vi "ZNA_setMarker.vi"(5 "Step_Freq(GHz)":dbl=0.5 format="%#_13g", 7 "Start_Freq(GHz)":dbl=26.5 format="%#_13g", 8 "error in":errorcluster, 9 "Simulation":bool, 10 "Markers_num":i32=11, 11 "VISA IN":refnum<visa-resource-name>="TCPIP0::192.168.100.12::inst0::INSTR") -> (0 "error out":errorcluster, 3 "Marker_array":dbl[](array[numeric]))   [LabVIEW 2023, in "R_S.lvlib"]
uses:
  R_S.lvlib
  CTL/RS_ZNA.ctl
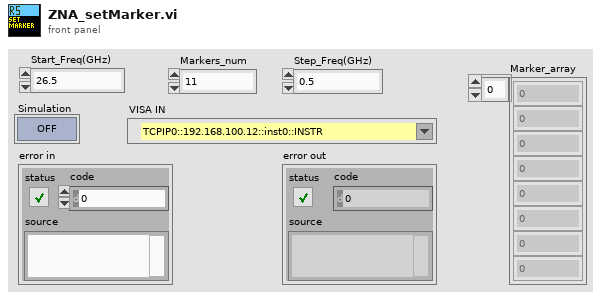
[diagram p1: front panel]
types:
  T1 = typedef "RS_ZNA.ctl" = enum16{"Init", "Close", "set_SweepPoint", "set_MeasFormat", "set_FreqStartStop", "set_MeasPAR_S", "set_MarkerON", "set_MarkerOFF", "set_MarkerFreq", "set_MarkerFormat", "set_TriggerSingle", "query_GainPhase"}
  T2 = cluster{"SweepPoints":i32, "StartFreq_GHz":dbl, "StopFreq_GHz":dbl, "S_Parameter":i32, "Marker_no.":i32, "Marker_Freq(GHz)":dbl}
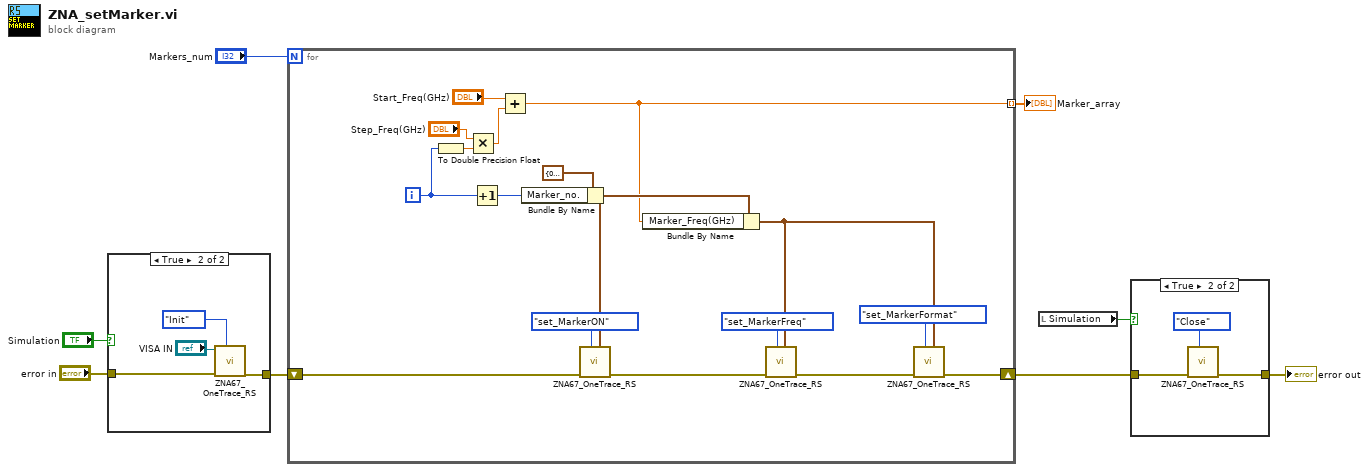
[diagram p0: block diagram]
diagram:
  n1 = case shown="True" "Simulation" {
    tunnel: "error in" -> [w9 w13]
    tunnel: [w9 w11] -> w7
    frame False {
    }
    frame True {
      n2 = call "ZNA67_OneTrace_RS.vi"("ZNA_Func."=RS_ZNA."Init", "error in"=w13, "VISA IN"="VISA IN") -> ("error out"=w11:errorcluster)  [unwired: 5 in, 3 out]
    }
  }
  n3 = for {
    N: "Markers_num" -> [_]
    shift-right: [w20] -> w6
    shift-left: w7 -> [w30]
    tunnel: [w18] -> w1 mode=indexing
    i -> [w28]
    n4 = To Double Precision Float(number=w28) -> (double precision float=w26:dbl)
    n5 = Multiply(x="Step_Freq(GHz)", y=w26) -> (x*y=w24:dbl)
    n6 = Increment(x=w28) -> (x+1=w22:i32)
    n7 = Add(x="Start_Freq(GHz)", y=w24) -> (x+y=w18:dbl)
    n8 = Bundle By Name(cluster=T2 {"SweepPoints"=0, "StartFreq_GHz"=0.0, "StopFreq_GHz"=0.0, "S_Parameter"=0, "Marker_no."=0, "Marker_Freq(GHz)"=0.0} ("ZNA_Parameters"), "Marker_no."=w22) -> (w23:T2)
    n9 = call "ZNA67_OneTrace_RS.vi"("ZNA_Parameters"=w23, "ZNA_Func."=RS_ZNA."set_MarkerON", "error in"=w30) -> ("error out"=w29:errorcluster)  [unwired: 5 in, 3 out]
    n10 = Bundle By Name(cluster=w23, "Marker_Freq(GHz)"=w18) -> (w19:T2)
    n11 = call "ZNA67_OneTrace_RS.vi"("ZNA_Parameters"=w19, "ZNA_Func."=RS_ZNA."set_MarkerFreq", "error in"=w29) -> ("error out"=w21:errorcluster)  [unwired: 5 in, 3 out]
    n12 = call "ZNA67_OneTrace_RS.vi"("ZNA_Parameters"=w19, "ZNA_Func."=RS_ZNA."set_MarkerFormat", "error in"=w21) -> ("error out"=w20:errorcluster)  [unwired: 5 in, 3 out]
  }
  "Marker_array" <- w1
  n13 = local read "Simulation"() -> (w2:bool)
  n14 = case shown="True" w2 {
    tunnel: w6 -> [w31 w34]
    tunnel: [w31 w33] -> w4
    frame False {
    }
    frame True {
      n15 = call "ZNA67_OneTrace_RS.vi"("ZNA_Func."=RS_ZNA."Close", "error in"=w34) -> ("error out"=w33:errorcluster)  [unwired: 6 in, 3 out]
    }
  }
  "error out" <- w4
